vi "Receive.vi"(7 "Device Address":u8, 8 "error in (no error)":errorcluster, 9 "eI2Cflags":T1 caption="I2C Flags" items=["None"=0, "START"=2, "REPEATED START"=3, "STOP"=4, "START AND STOP"=6], 10 "Bytes To Read":u32, 11 "II2COUSB in":refnum<class "II2COUSB.lvclass">) -> (0 "error out":errorcluster, 1 "Status":string, 2 "Buffer":u8[](array[numeric]), 3 "II2COUSB out":refnum<class "II2COUSB.lvclass">, 5 "Byte Returned":u32)   [LabVIEW 2020, in "II2COUSB.lvlib" / "II2COUSB.lvclass"]
doc: "Receive Data"
uses:
  II2COUSB.lvclass
  TypeDef/I2CFlags.ctl
  TypeDef/II2COUSB_typedef.lvlib
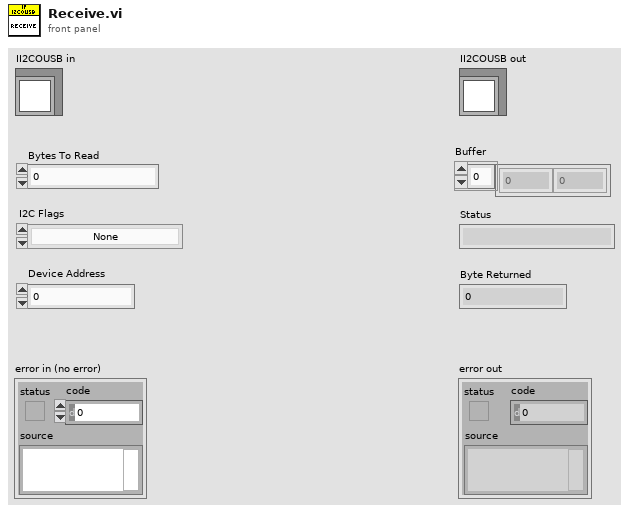
[diagram p1: front panel]
types:
  T1 = typedef "II2COUSB_typedef.lvlib/I2CFlags.ctl" = u8
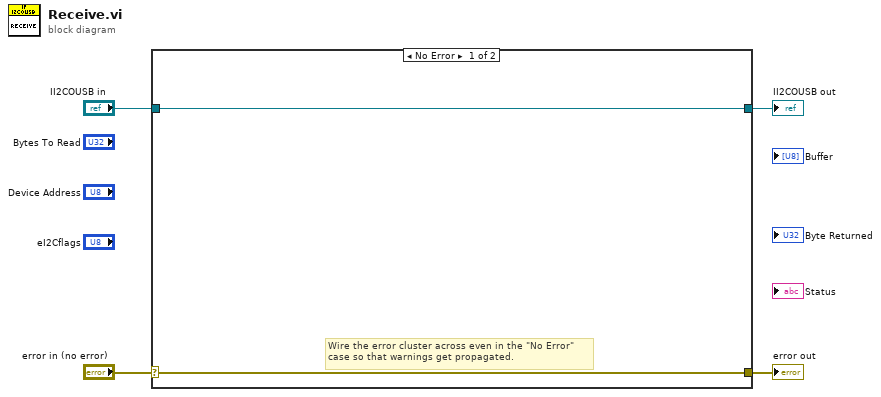
[diagram p0: block diagram]
diagram:
  n1 = case shown="No Error" "error in (no error)" {
    selector: "error in (no error)" -> [w5 w8]
    tunnel: [w5 w8] -> w3
    tunnel: [w6 w7] -> w1
    tunnel: "II2COUSB in" -> [w6 w7]
    frame No Error {
      # "Wire the error cluster across even in the \"No Error\"\ncase so that warnings get propagated."
    }
    frame Error {
    }
  }
  "error out" <- w3
  "II2COUSB out" <- w1
